vi "Draw Simple Skeleton Picture.vi"(6 "Color":u32(colorbox)=1965842, 7 "Dot Size":i32=10, 8 "Bounds":T1, 10 "Simple Skeleton":T4, 11 "new picture in":picture) -> (3 "new picture out":picture)   [LabVIEW 2012]
uses:
  <vilib>/addons/Kinect/SkeletonVertexTrackState.ctl
  <vilib>/addons/Kinect/SkeletonTrackState.ctl
  <vilib>/Utility/miscctls.llb/LVBoundsTypeDef.ctl
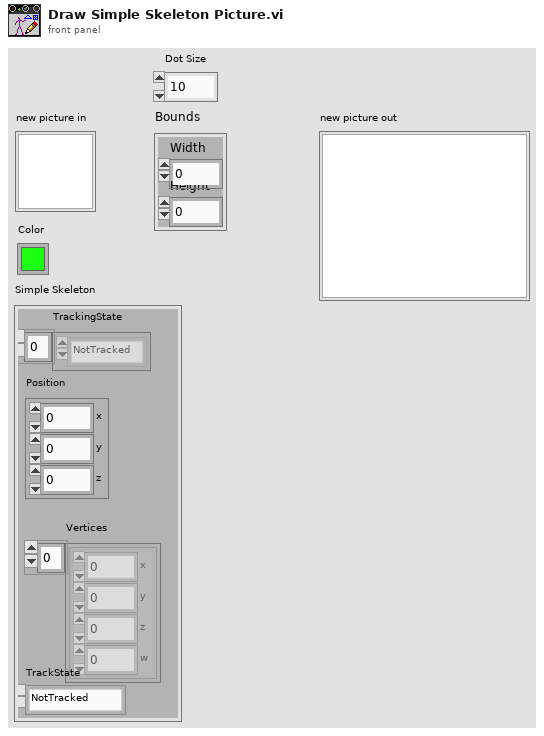
[diagram p1: front panel]
types:
  T1 = typedef "LVBoundsTypeDef.ctl" = cluster{"Width":u32, "Height":u32}
  T2 = typedef "SkeletonVertexTrackState.ctl" = enum32{"NotTracked", "Inferred", "Tracked"}
  T3 = typedef "SkeletonTrackState.ctl" = enum32{"NotTracked", "PositionOnly", "Tracked"}
  T4 = cluster{"TrackingState":T2[], "Position":cluster{"x":sgl, "y":sgl, "z":sgl}, "Vertices":cluster{"x":sgl, "y":sgl, "z":sgl, "w":sgl}[], "TrackState":T3}
  T5 = typedef "Vector4.ctl" = cluster{"x":sgl, "y":sgl, "z":sgl, "w":sgl}
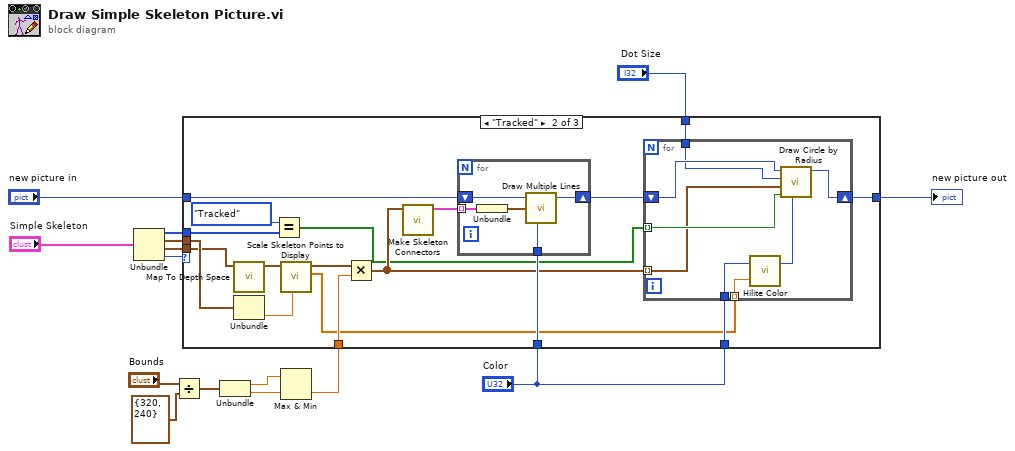
[diagram p0: block diagram]
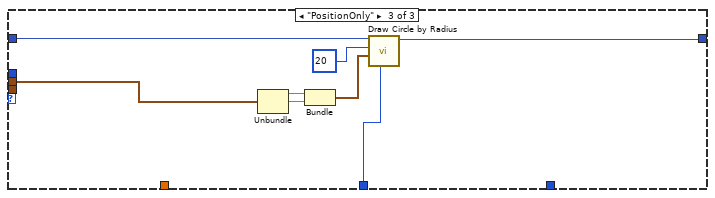
[diagram p3: hidden frame]
diagram:
  n1 = Unbundle("Simple Skeleton") -> ("TrackingState"=w12:T2[], "Position"=w9:cluster{"x":sgl, "y":sgl, "z":sgl}, "Vertices"=w7:cluster{"x":sgl, "y":sgl, "z":sgl, "w":sgl}[], "TrackState"=w8:T3)
  n2 = Divide(x="Bounds", y=T1 {"Width"=320, "Height"=240} ("Bounds")) -> (x/y=w4:cluster{"Width":dbl, "Height":dbl})
  n3 = Unbundle(w4) -> ("Width"=w2:dbl, "Height"=w3:dbl)
  n4 = Max & Min(x=w2, y=w3) -> (min(x,y)=w1:dbl)  [unwired: 1 out]
  n5 = case shown="\"Tracked\"" w8 {
    tunnel: "Color" -> [_ w34 _]
    tunnel: "Dot Size" -> [_ w33 _]
    tunnel: [w16 w32 w54] -> w14
    tunnel: w1 -> [_ w30 _]
    tunnel: "new picture in" -> [w16 w28 w55]
    tunnel: "Color" -> [_ w27 w52]
    tunnel: w9 -> [_ w22 w48]
    tunnel: w12 -> [_ w20 _]
    tunnel: w7 -> [_ w17 _]
    frame "NotTracked", Default {
    }
    frame "Tracked" {
      n6 = call <vilib>:"Map To Depth Space.vi"("Vertices in"=w17) -> ("Vertices out"=w23:T5[])  [unwired: 10 in]
      n7 = Unbundle(w22) -> ("z"=w21:sgl)  [unwired: 2 out]
      n8 = Equal?(x=SkeletonVertexTrackState."Tracked", y=w20) -> (x = y?=w18:bool[])
      n9 = call <vilib>:"Scale Skeleton Points to Display.vi"("Mean Distance"=w21, "Vertices out"=w23) -> ("Z Intensities"=w25:sgl[], "Image Points"=w24:cluster{sgl, sgl}[])  [unwired: 8 in]
      n10 = Multiply(x=w24, y=w30) -> (x*y=w26:cluster{dbl, dbl}[])
      n11 = call <vilib>:"Make Skeleton Connectors.vi"("Joints"=w26) -> ("Connectors"=w29:cluster{cluster{sgl, sgl}[]}[])  [unwired: 10 in]
      n12 = for {
        tunnel: w29 -> [w38] mode=indexing
        shift-right: [w39] -> w31
        shift-left: w28 -> [w36]
        tunnel: w27 -> [w35]
        n13 = Unbundle(w38) -> (w37:cluster{sgl, sgl}[])
        n14 = call <vilib>:"Draw Multiple Lines.vi"("picture"=w36, "line endpoints"=w37, "color(black)"=w35) -> ("new picture"=w39:picture)  [unwired: 6 in]
      }
      n15 = for {
        shift-right: [w46] -> w32
        shift-left: w31 -> [w47]
        tunnel: w26 -> [w40] mode=indexing
        tunnel: w34 -> [w45]
        tunnel: w33 -> [w43]
        tunnel: w25 -> [w42] mode=indexing
        tunnel: w18 -> [w41] mode=indexing
        n16 = call <vilib>:"Hilite Color.vi"("Percentage(30)"=w42, "Color In"=w45) -> ("Hilite"=w44:u32)  [unwired: 1 out]
        n17 = call <vilib>:"Draw Circle by Radius.vi"("color(black)"=w44, "fill?(F)"=w41, "pixel center"=w40, "radius"=w43, "picture"=w47) -> ("new picture"=w46:picture)  [unwired: 6 in]
      }
    }
    frame "PositionOnly" {
      n18 = Unbundle(w48) -> ("x"=w50:sgl, "y"=w51:sgl)  [unwired: 1 out]
      n19 = Bundle("x"=w50, "y"=w51) -> (w49:cluster{"x":sgl, "y":sgl})  [unwired: 1 in]
      n20 = call <vilib>:"Draw Circle by Radius.vi"("color(black)"=w52, "pixel center"=w49, "radius"=20, "picture"=w55) -> ("new picture"=w54:picture)  [unwired: 7 in]
    }
  }
  "new picture out" <- w14
